vi "oa_TV Differentiator (NChan).vi"(5 "reset? (False)":bool, 8 "error in (no error)":errorcluster, 10 "delta X":dbl[](array[numeric])=[1.0, 1.0, 1.0] format="%.2f", 11 "Y[n]":cluster{dbl[]}[](array[cluster]) {"?" format="%.2f"}) -> (0 "error out":errorcluster, 1 "Delay":dbl[](array[numeric]), 2 "X[n]":cluster{dbl[]}[](array[cluster]), 3 "dY[n]/dX[n]":cluster{dbl[]}[](array[cluster]))   [LabVIEW 2017, in "SoundVib_Torsional.lvlib"]
uses:
  <vilib>/addons/Sound and Vibration/Order Analysis/Torsional Vibration/SoundVib_Torsional.lvlib
  <vilib>/Analysis/3filter.llb/FIR Filter with I.C. (DBL).vi
  <vilib>/Analysis/NI_AALBase.lvlib
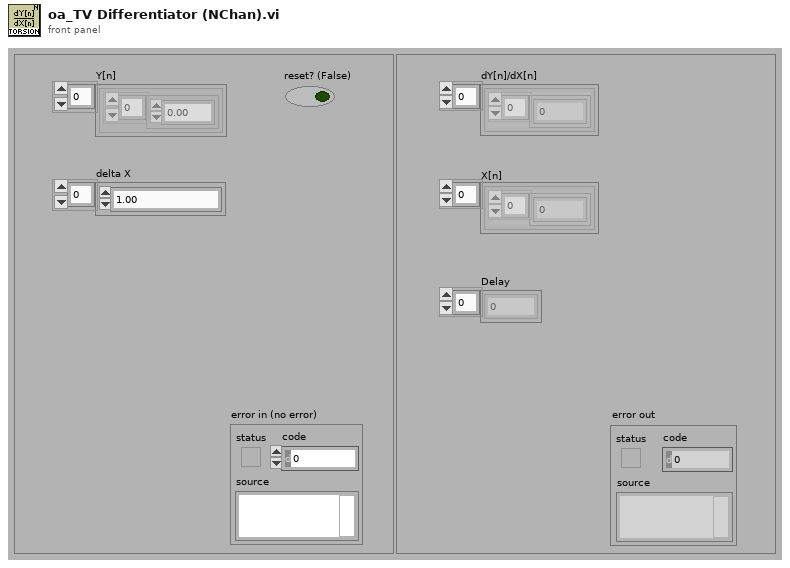
[diagram p1: front panel]
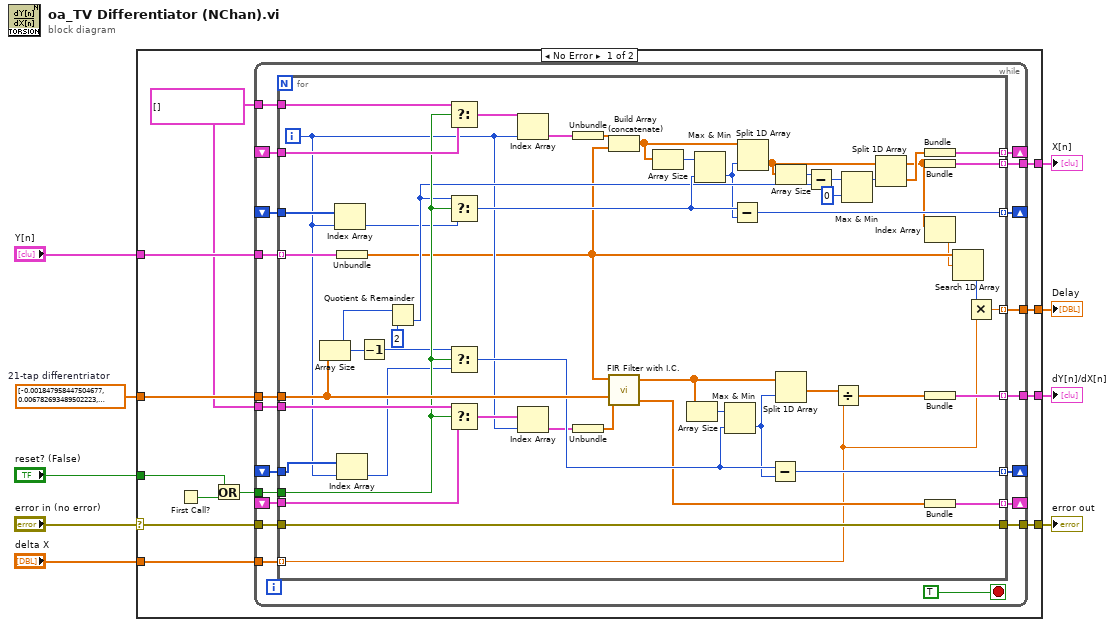
[diagram p0: block diagram]
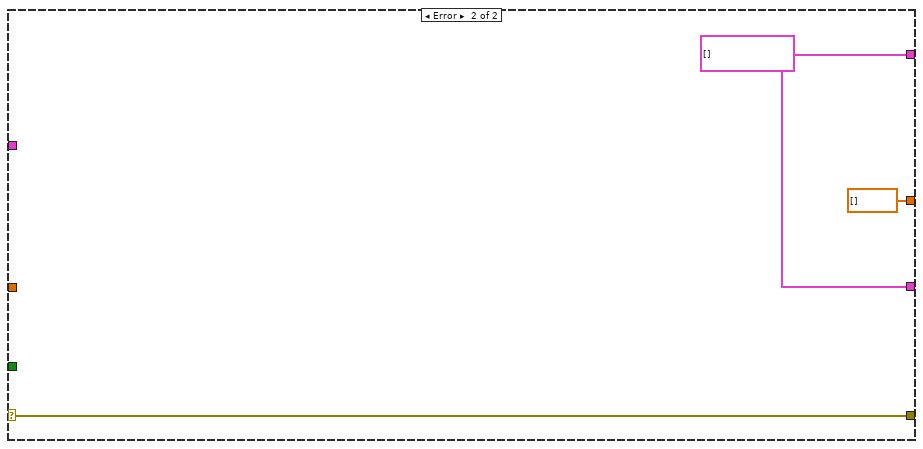
[diagram p2: hidden frame]
diagram:
  w2 = dbl[] [-0.001847958447504677, 0.006782693489502223, -0.015759314785292692, 0.03157696398653407, -0.05723345514019107, 0.09716912388312568, -0.15901162473423236, 0.2593879138454093, -0.4476586474107506, 0.9725301910180191, 0.0, -0.9725301910180191, 0.4476586474107506, -0.2593879138454093, 0.15901162473423236, -0.09716912388312568, 0.05723345514019107, -0.03157696398653407, 0.015759314785292692, -0.006782693489502223, 0.001847958447504677]  # 21-tap differentriator
  n1 = case shown="No Error" "error in (no error)" {
    selector: "error in (no error)" -> [w21 w96]
    tunnel: [w19 w96] -> w7
    tunnel: "Y[n]" -> [w17 _]
    tunnel: w2 -> [w20 _]
    tunnel: "reset? (False)" -> [w16 _]
    tunnel: [w18 w95] -> w5
    tunnel: [w13 w95] -> w4
    tunnel: "delta X" -> [w12 _]
    tunnel: [w10 dbl[] []] -> w1
    frame No Error {
      w11 = cluster{dbl[]}[] []
      n2 = First Call?() -> (First Call?: T/F=w14:bool)
      n3 = Or(x=w16, y=w14) -> (x .or. y?=w15:bool)
      n4 = while {
        tunnel: w21 -> [w41]
        tunnel: w20 -> [w32]
        shift-right: [w23] -> _
        shift-left: _ -> [w35]
        shift-right: [w24] -> _
        shift-left: _ -> [w39]
        shift-right: [w30] -> _
        shift-left: _ -> [w27]
        tunnel: w15 -> [w37]
        tunnel: w11 -> [w38]
        shift-right: [w29] -> _
        shift-left: _ -> [w28]
        tunnel: w11 -> [w36]
        tunnel: w17 -> [w31]
        tunnel: [w34] -> w19
        tunnel: [w33] -> w18
        tunnel: [w26] -> w13
        tunnel: w12 -> [w25]
        tunnel: [w22] -> w10
        stop <- TRUE stop-if-true
        n5 = for {
          tunnel: w41 -> [w85]
          tunnel: w32 -> [w80]
          tunnel: [w93] -> w30 mode=indexing
          tunnel: [w92] -> w29 mode=indexing
          tunnel: w27 -> [w53]
          tunnel: [w60] -> w24 mode=indexing
          tunnel: w39 -> [w90]
          tunnel: w38 -> [w89]
          tunnel: w37 -> [w79]
          tunnel: w36 -> [w88]
          tunnel: w35 -> [w87]
          tunnel: w31 -> [w82] mode=indexing
          tunnel: [w58] -> w23 mode=indexing
          tunnel: [w85] -> w34
          tunnel: [w84] -> w33 mode=indexing
          tunnel: [w83] -> w26 mode=indexing
          tunnel: w28 -> [w51]
          tunnel: w25 -> [w43] mode=indexing
          tunnel: [w42] -> w22 mode=indexing
          i -> [w50]
          n6 = Array Size(array=w80) -> (size(s)=w48:i32)
          n7 = Index Array(array=w53, index=w50) -> (element=w52:i32)
          n8 = Unbundle(w82) -> (w46:dbl[])
          n9 = Index Array(array=w51, index=w50) -> (element=w49:i32)
          n10 = Decrement(x=w48) -> (x-1=w76:i32)
          n11 = Quotient & Remainder(x=w48, y=2) -> (floor(x/y)=w77:i32)  [unwired: 1 out]
          n12 = Select(t=w89, s=w79, f=w90) -> (s? t:f=w91:cluster{dbl[]}[])
          n13 = Select(t=w77, s=w79, f=w52) -> (s? t:f=w78:i32)
          n14 = Select(t=w76, s=w79, f=w49) -> (s? t:f=w75:i32)
          n15 = Select(t=w88, s=w79, f=w87) -> (s? t:f=w86:cluster{"Final X Conditions":dbl[]}[])
          n16 = Index Array(array=w91, index=w50) -> (element=w57:cluster{dbl[]})
          n17 = Index Array(array=w86, index=w50) -> (element=w55:cluster{"Final X Conditions":dbl[]})
          n18 = Unbundle(w57) -> (w56:dbl[])
          n19 = Unbundle(w55) -> ("Final X Conditions"=w54:dbl[])
          n20 = Build Array (concatenate)(w56, w46) -> (w65:dbl[])
          n21 = call-poly <vilib>:"FIR Filter with I.C..vi"("Initial X Conditions"=w54, "FIR Coefficients"=w80, "X"=w46) -> ("Final X Conditions"=w59:dbl[], "Filtered X"=w64:dbl[])  [unwired: 5 in, 1 out]
          n22 = Array Size(array=w65) -> (size(s)=w74:i32)
          n23 = Array Size(array=w64) -> (size(s)=w68:i32)
          n24 = Max & Min(x=w74, y=w78) -> (min(x,y)=w73:i32)  [unwired: 1 out]
          n25 = Max & Min(x=w68, y=w75) -> (min(x,y)=w67:i32)  [unwired: 1 out]
          n26 = Subtract(x=w78, y=w73) -> (x-y=w93:i32)
          n27 = Split 1D Array(array=w65, index=w73) -> (second subarray=w72:dbl[])  [unwired: 1 out]
          n28 = Subtract(x=w75, y=w67) -> (x-y=w92:i32)
          n29 = Array Size(array=w72) -> (size(s)=w71:i32)
          n30 = Split 1D Array(array=w64, index=w67) -> (second subarray=w63:dbl[])  [unwired: 1 out]
          n31 = Subtract(x=w71, y=w77) -> (x-y=w70:i32)
          n32 = Divide(x=w63, y=w43) -> (x/y=w62:dbl[])
          n33 = Max & Min(x=w70, y=0) -> (max(x,y)=w66:i32)  [unwired: 1 out]
          n34 = Split 1D Array(array=w72, index=w66) -> (first subarray=w47:dbl[], second subarray=w61:dbl[])
          n35 = Bundle(w61) -> (w60:cluster{dbl[]})  [unwired: 1 in]
          n36 = Bundle(w47) -> (w84:cluster{dbl[]})  [unwired: 1 in]
          n37 = Index Array(array=w47) -> (element=w45:dbl)  [unwired: 1 in]
          n38 = Bundle(w62) -> (w83:cluster{dbl[]})  [unwired: 1 in]
          n39 = Bundle("Final X Conditions"=w59) -> (w58:cluster{"Final X Conditions":dbl[]})  [unwired: 1 in]
          n40 = Search 1D Array(1D array=w46, element=w45) -> (index of element=w44:i32)  [unwired: 1 in]
          n41 = Multiply(x=w44, y=w43) -> (x*y=w42:dbl)
        }
      }
    }
    frame Error {
      w95 = cluster{dbl[]}[] []
    }
  }
  "error out" <- w7
  "X[n]" <- w5
  "dY[n]/dX[n]" <- w4
  "Delay" <- w1
